vi "onValidateExpression.vi"(8 "error in (no error)":errorcluster, 10 "Expression":string, 11 "Cron.Quartz in":refnum<class "Cron.Quartz.lvclass">) -> (0 "error out":errorcluster, 1 "valid?":bool, 2 "Validated Expression":string, 3 "Cron.Quartz out":refnum<class "Cron.Quartz.lvclass">)   [LabVIEW 2013, in "openCron.lvlib" / "Cron.Quartz.lvclass"]
uses:
  Cron.Quartz.lvclass
  Cron/Cron.lvclass
  <vilib>/regexp/Match Regular Expression.xnode
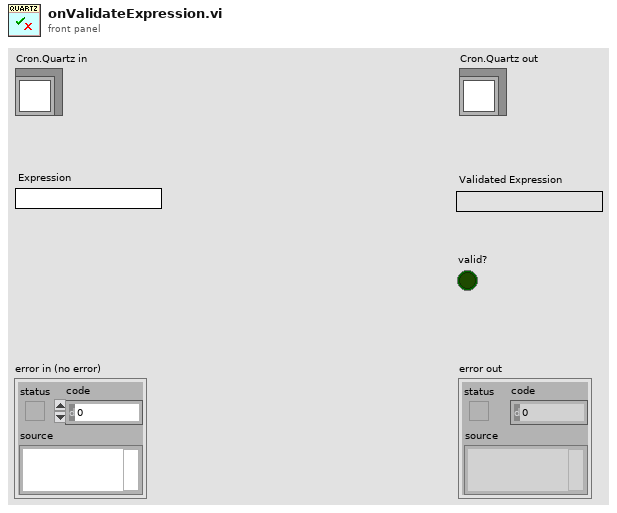
[diagram p1: front panel]
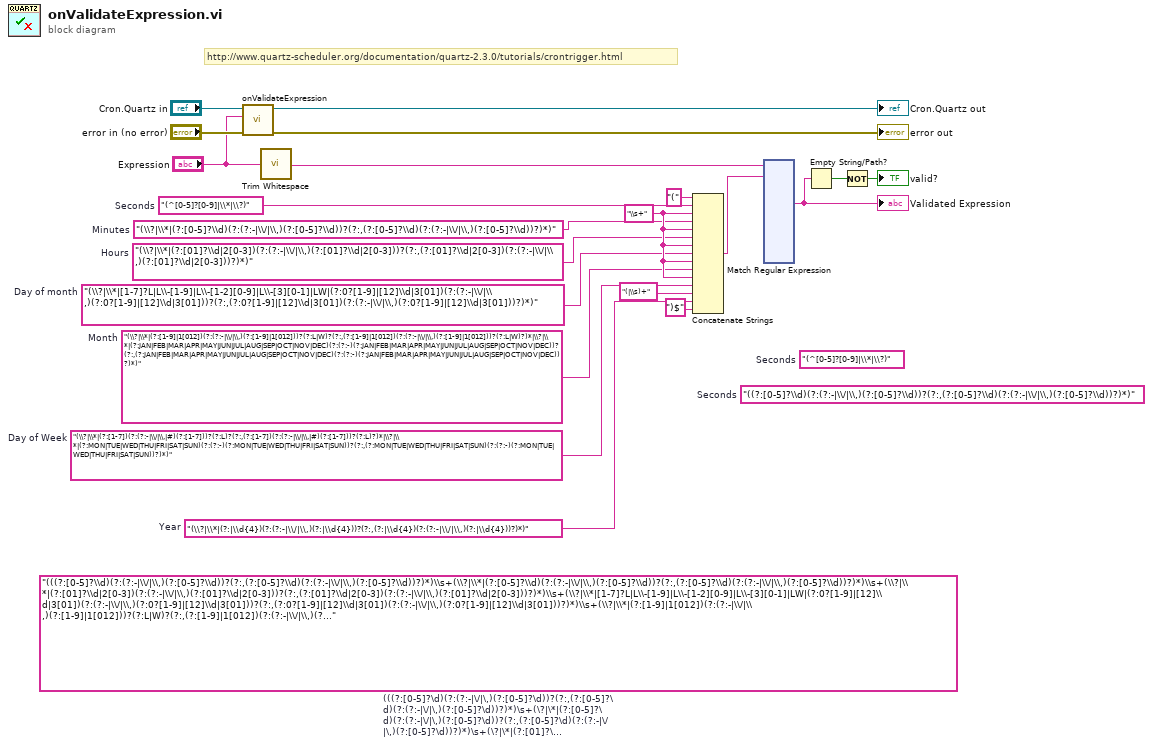
[diagram p0: block diagram]
diagram:
  (unwired) "(^[0-5]?[0-9]|\\*|\\?)"  # Seconds
  (unwired) "((?:[0-5]?\\d)(?:(?:-|\\/|\\,)(?:[0-5]?\\d))?(?:,(?:[0-5]?\\d)(?:(?:-|\\/|\\,)(?:[0-5]?\\d))?)*)"  # Seconds
  w2 = "(\\?|\\*|(?:|\\d{4})(?:(?:-|\\/|\\,)(?:|\\d{4}))?(?:,(?:|\\d{4})(?:(?:-|\\/|\\,)(?:|\\d{4}))?)*)"  # Year
  w4 = "(\\?|\\*|(?:[1-9]|1[012])(?:(?:-|\\/|\\,)(?:[1-9]|1[012]))?(?:L|W)?(?:,(?:[1-9]|1[012])(?:(?:-|\\/|\\,)(?:[1-9]|1[012]))?(?:L|W)?)*|\\?|\\*|(?:JAN|FEB|MAR|APR|MAY|JUN|JUL|AUG|SEP|OCT|NOV|DEC)(?:(?:-)(?:JAN|FEB|MAR|APR|MAY|JUN|JUL|AUG|SEP|OCT|NOV|DEC))?(?:,(?:JAN|FEB|MAR|APR|MAY|JUN|JUL|AUG|SEP|OCT|NOV|DEC)(?:(?:-)(?:JAN|FEB|MAR|APR|MAY|JUN|JUL|AUG|SEP|OCT|NOV|DEC))?)*)"  # Month
  w3 = "(\\?|\\*|[1-7]?L|L\\-[1-9]|L\\-[1-2][0-9]|L\\-[3][0-1]|LW|(?:0?[1-9]|[12]\\d|3[01])(?:(?:-|\\/|\\,)(?:0?[1-9]|[12]\\d|3[01]))?(?:,(?:0?[1-9]|[12]\\d|3[01])(?:(?:-|\\/|\\,)(?:0?[1-9]|[12]\\d|3[01]))?)*)"  # Day of month
  w5 = "(\\?|\\*|(?:[1-7])(?:(?:-|\\/|\\,|#)(?:[1-7]))?(?:L)?(?:,(?:[1-7])(?:(?:-|\\/|\\,|#)(?:[1-7]))?(?:L)?)*|\\?|\\*|(?:MON|TUE|WED|THU|FRI|SAT|SUN)(?:(?:-)(?:MON|TUE|WED|THU|FRI|SAT|SUN))?(?:,(?:MON|TUE|WED|THU|FRI|SAT|SUN)(?:(?:-)(?:MON|TUE|WED|THU|FRI|SAT|SUN))?)*)"  # Day of Week
  w7 = "(\\?|\\*|(?:[0-5]?\\d)(?:(?:-|\\/|\\,)(?:[0-5]?\\d))?(?:,(?:[0-5]?\\d)(?:(?:-|\\/|\\,)(?:[0-5]?\\d))?)*)"  # Minutes
  w8 = "(^[0-5]?[0-9]|\\*|\\?)"  # Seconds
  w12 = "\\s+"
  w6 = "(\\?|\\*|(?:[01]?\\d|2[0-3])(?:(?:-|\\/|\\,)(?:[01]?\\d|2[0-3]))?(?:,(?:[01]?\\d|2[0-3])(?:(?:-|\\/|\\,)(?:[01]?\\d|2[0-3]))?)*)"  # Hours
  (unwired) "(((?:[0-5]?\\d)(?:(?:-|\\/|\\,)(?:[0-5]?\\d))?(?:,(?:[0-5]?\\d)(?:(?:-|\\/|\\,)(?:[0-5]?\\d))?)*)\\s+(\\?|\\*|(?:[0-5]?\\d)(?:(?:-|\\/|\\,)(?:[0-5]?\\d))?(?:,(?:[0-5]?\\d)(?:(?:-|\\/|\\,)(?:[0-5]?\\d))?)*)\\s+(\\?|\\*|(?:[01]?\\d|2[0-3])(?:(?:-|\\/|\\,)(?:[01]?\\d|2[0-3]))?(?:,(?:[01]?\\d|2[0-3])(?:(?:-|\\/|\\,)(?:[01]?\\d|2[0-3]))?)*)\\s+(\\?|\\*|[1-7]?L|L\\-[1-9]|L\\-[1-2][0-9]|L\\-[3][0-1]|LW|(?:0?[1-9]|[12]\\d|3[01])(?:(?:-|\\/|\\,)(?:0?[1-9]|[12]\\d|3[01]))?(?:,(?:0?[1-9]|[12]\\d|3[01])(?:(?:-|\\/|\\,)(?:0?[1-9]|[12]\\d|3[01]))?)*)\\s+(\\?|\\*|(?:[1-9]|1[012])(?:(?:-|\\/|\\,)(?:[1-9]|1[012]))?(?:L|W)?(?:,(?:[1-9]|1[012])(?:(?:-|\\/|\\,)(?:[1-9]|1[012]))?(?:L|W)?)*|\\?|\\*|(?:JAN|FEB|MAR|APR|MAY|JUN|JUL|AUG|SEP|OCT|NOV|DEC)(?:(?:-)(?:JAN|FEB|MAR|APR|MAY|JUN|JUL|AUG|SEP|OCT|NOV|DEC))?(?:,(?:JAN|FEB|MAR|APR|MAY|JUN|JUL|AUG|SEP|OCT|NOV|DEC)(?:(?:-)(?:JAN|FEB|MAR|APR|MAY|JUN|JUL|AUG|SEP|OCT|NOV|DEC))?)*)\\s+(\\?|\\*|(?:[1-7])(?:(?:-|\\/|\\,|#)(?:[1-7]))?(?:L)?(?:,(?:[1-7])(?:(?:-|\\/|\\,|#)(?:[1-7]))?(?:L)?)*|\\?|\\*|(?:MON|TUE|WED|THU|FRI|SAT|SUN)(?:(?:-)(?:MON|TUE|WED|THU|FRI|SAT|SUN))?(?:,(?:MON|TUE|WED|THU|FRI|SAT|SUN)(?:(?:-)(?:MON|TUE|WED|THU|FRI|SAT|SUN))?)*)(|\\s)+(\\?|\\*|(?:|\\d{4})(?:(?:-|\\/|\\,)(?:|\\d{4}))?(?:,(?:|\\d{4})(?:(?:-|\\/|\\,)(?:|\\d{4}))?)*))$"  # (((?:[0-5]?\d)(?:(?:-|\/|\,)(?:[0-5]?\d))?(?:,(?:[0-5]?\d)(?:(?:-|\/|\,)(?:[0-5]?\d))?)*)\s+(\?|\*|(?:[0-5]?\d)(?:(?:-|\/|\,)(?:[0-5]?\d))?(?:,(?:[0-5]?\d)(?:(?:-|\/|\,)(?:[0-5]?\d))?)*)\s+(\?|\*|(?:[01]?\d|2[0-3])(?:(?:-|\/|\,)(?:[01]?\d|2[0-3]))?(?:,(?:[01]?\d|2[0-3])(?:(?:-|\/|\,)(?:[01]?\d|2[0-3]))?)*)\s+(\?|\*|[1-7]?L|L\-[1-9]|L\-[1-2][0-9]|L\-[3][0-1]|LW|(?:0?[1-9]|[12]\d|3[01])(?:(?:-|\/|\,)(?:0?[1-9]|[12]\d|3[01]))?(?:,(?:0?[1-9]|[12]\d|3[01])(?:(?:-|\/|\,)(?:0?[1-9]|[12]\d|3[01]))?)*)\s+(\?|\*|(?:[1-9]|1[012])(?:(?:-|\/|\,)(?:[1-9]|1[012]))?(?:L|W)?(?:,(?:[1-9]|1[012])(?:(?:-|\/|\,)(?:[1-9]|1[012]))?(?:L|W)?)*|\?|\*|(?:JAN|FEB|MAR|APR|MAY|JUN|JUL|AUG|SEP|OCT|NOV|DEC)(?:(?:-)(?:JAN|FEB|MAR|APR|MAY|JUN|JUL|AUG|SEP|OCT|NOV|DEC))?(?:,(?:JAN|FEB|MAR|APR|MAY|JUN|JUL|AUG|SEP|OCT|NOV|DEC)(?:(?:-)(?:JAN|FEB|MAR|APR|MAY|JUN|JUL|AUG|SEP|OCT|NOV|DEC))?)*)\s+(\?|\*|(?:[1-7])(?:(?:-|\/|\,|#)(?:[1-7]))?(?:L)?(?:,(?:[1-7])(?:(?:-|\/|\,|#)(?:[1-7]))?(?:L)?)*|\?|\*|(?:MON|TUE|WED|THU|FRI|SAT|SUN)(?:(?:-)(?:MON|TUE|WED|THU|FRI|SAT|SUN))?(?:,(?:MON|TUE|WED|THU|FRI|SAT|SUN)(?:(?:-)(?:MON|TUE|WED|THU|FRI|SAT|SUN))?)*)(|\s)+(\?|\*|(?:|\d{4})(?:(?:-|\/|\,)(?:|\d{4}))?(?:,(?:|\d{4})(?:(?:-|\/|\,)(?:|\d{4}))?)*))$
  # "http://www.quartz-scheduler.org/documentation/quartz-2.3.0/tutorials/crontrigger.html"
  n1 = call-parent "onValidateExpression.vi"("error in (no error)"="error in (no error)", "Expression"="Expression", "Cron in"="Cron.Quartz in") -> ("error out"=→"error out":errorcluster, "Cron out"=→"Cron.Quartz out":refnum<class "Cron.Quartz.lvclass">)  [unwired: 5 in, 2 out]
  n2 = call <vilib>:"Trim Whitespace.vi"("string"="Expression") -> ("trimmed string"=w16:string)  [unwired: 1 in]
  n3 = Concatenate Strings("(", w8, w12, w7, w12, w6, w12, w3, w12, w4, w12, w5, "(|\\s)+", w2, ")$") -> (w1:string)
  n4 = xnode "Match Regular Expression"("input string"=w16, "regular expression"=w1) -> ("submatch 1"=w15:string)  [unwired: 4 in, 12 out]
  "Validated Expression" <- w15
  n5 = Empty String/Path?(string/path=w15) -> (empty?=w14:bool)
  n6 = Not(x=w14) -> (.not. x?=→"valid?":bool)
